vi "Initialize IR GALVO DAQ (SubVI).vi"() -> (3 "Refnum out":refnum<k21>)   [LabVIEW 2020]
uses:
  <vilib>/DAQmx/configure/timing.llb/DAQmx Timing (Sample Clock).vi
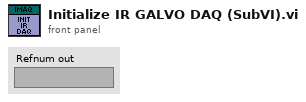
[diagram p1: front panel]
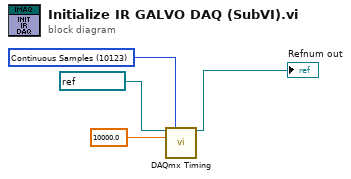
[diagram p0: block diagram]
diagram:
  w1 = 10123 items=["Finite Samples"=10178, "Continuous Samples"=10123, "Hardware Timed Single Point"=12522] ("sample mode")
  n1 = call-poly <vilib>:"DAQmx Timing.vi"("task/channels in"=refnum<k21> "GALVO" ("DAQmx Task Name"), "sample mode"=w1, "rate"=10000.0 ("Rate")) -> ("task out"=→"Refnum out":refnum<k21>)  [unwired: 11 in, 1 out]
